vi "Emballage_NoCmd_NomProduit.vi"(8 "Error in":errorcluster caption="Error in (no error)", 11 "NO_CDEVAL":string="6340/07-02.01.01") -> (0 "Error out":errorcluster, 3 "Produit":string)   [LabVIEW 2020]
uses:
  Modules/FS/60_FS_Controles/60_FS_SetGet.ctl
  <vilib>/addons/database/Connection.llb/DB Tools Open Connec (Path).vi
  <vilib>/addons/database/Connection.llb/Conn Execute.vi
  <vilib>/addons/database/Recordset.llb/Rec Fetch Recordset Data (R).vi
  <vilib>/addons/database/Recordset.llb/Rec Destroy - Connection.vi
  <vilib>/addons/database/NI_Database_API.lvlib
panel:
  out "données 2":string[][](array[string])
  out "ID_ARTICLE_GPAO":string
  out "Donnees":string[][](array[string])
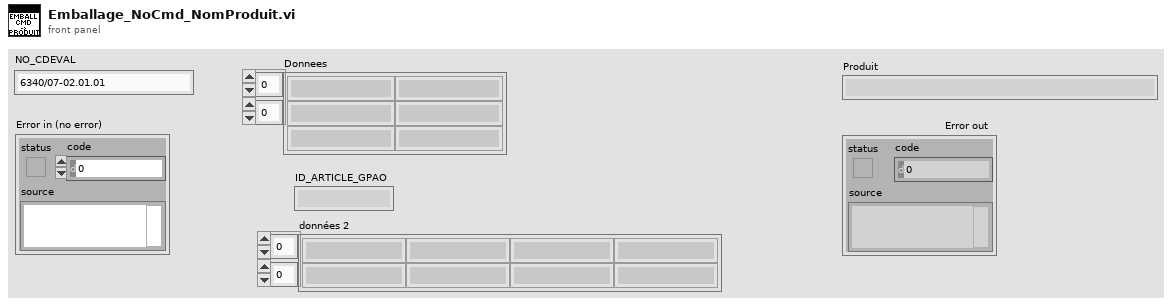
[diagram p1: front panel]
types:
  T1 = typedef "60_FS_SetGet.ctl" = enum16{"set", "get"}
  T2 = typedef "60_FS_CLT_Chemins.ctl" = cluster{"Racine_local":path, "Racine_reseau":path, "Racine_Support_Application":path, "Fichier_Journalisation":path, "Connexion_BDD_VSX":path, "Connexion_BDD_PLZ":path}
  T3 = typedef "NI_Database_API.lvlib/Conn ObjectReference.ctl" = refnum<k1>
  T4 = typedef "NI_Database_API.lvlib/Rec ObjectReference.ctl" = refnum<k1>
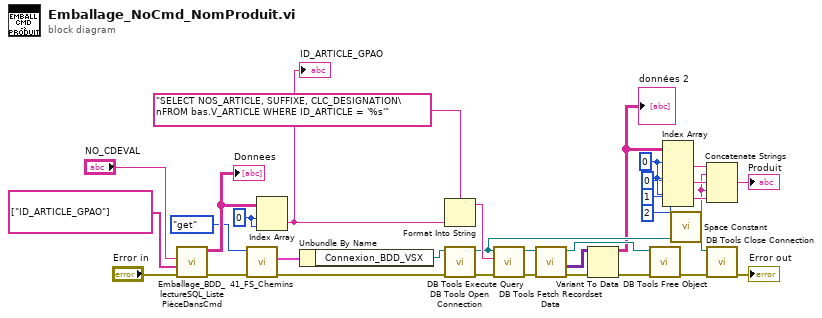
[diagram p0: block diagram]
diagram:
  w9 = 0 ("indice (ligne)")
  w29 = 0 ("indice (ligne)")
  n1 = call "Emballage_BDD_lectureSQL_Liste PièceDansCmd.vi"("Error in"="Error in", "Colonnes"=string[] ["ID_ARTICLE_GPAO"], "NO_CDEVAL"="NO_CDEVAL") -> ("Error out"=w12:errorcluster, "Donnees"=w30:string[][])  [unwired: 4 in, 3 out]
  "Donnees" <- w30
  n2 = call "41_FS_Chemins.vi"("error in (no error)"=w12, "SetGet"=60_FS_SetGet."get") -> ("error out"=w21:errorcluster, "CLT_Chemins_out"=w20:T2)  [unwired: 8 in]
  n3 = Index Array(array=w30, index (row)=w29, index (col)=w29) -> (element=w14:string)
  "ID_ARTICLE_GPAO" <- w14
  n4 = Unbundle By Name(w20) -> ("Connexion_BDD_VSX"=w28:path)
  n5 = Format Into String(format string="SELECT NOS_ARTICLE, SUFFIXE, CLC_DESIGNATION\nFROM bas.V_ARTICLE WHERE ID_ARTICLE = '%s'" ("SQL query"), w14) -> (resulting string=w15:string)  [unwired: 2 in, 1 out]
  n6 = call-poly <vilib>:"DB Tools Open Connection.vi"("error in (no error)"=w21, "connection information"=w28) -> ("error out"=w18:errorcluster, "connection reference"=w13:T3)  [unwired: 6 in]
  n7 = call-poly <vilib>:"DB Tools Execute Query.vi"("error in (no error)"=w18, "SQL query"=w15, "connection reference"=w13) -> ("error out"=w22:errorcluster, "recordset reference"=w23:T4)  [unwired: 5 in]
  n8 = call-poly <vilib>:"DB Tools Fetch Recordset Data.vi"("error in (no error)"=w22, "recordset reference"=w23) -> ("error out"=w25:errorcluster, "recordset data"=w24:variant[][], "recordset reference out"=w17:T4)  [unwired: 3 in]
  n9 = Variant To Data(error in=w25, Variant=w24) -> (data=w10:string[][], error out=w26:errorcluster)  [unwired: 1 in]
  "données 2" <- w10
  n10 = call-poly <vilib>:"DB Tools Free Object.vi"("error in (no error)"=w26, "recordset reference"=w17) -> ("error out"=w27:errorcluster)  [unwired: 8 in, 1 out]
  n11 = Index Array(array=w10, index (row) #1=w9, index (col) #1=0 ("indice désactivé (col)"), index (row) #2=w9, index (col) #2=1 ("indice désactivé (col)"), index (row) #3=w9, index (col) #3=2 ("indice désactivé (col)")) -> (element #1=w6:string, element #2=w8:string, element #3=w5:string)
  n12 = call <vilib>:"Space Constant.vi"() -> ("String"=w4:string)
  n13 = Concatenate Strings(w6, w4, w8, w4, w5) -> (→"Produit":string)
  n14 = call <vilib>:"DB Tools Close Connection.vi"("error in (no error)"=w27, "connection reference"=w13) -> ("error out"=→"Error out":errorcluster)  [unwired: 5 in]
